vi "FPGA.vi"() -> ()   [LabVIEW 2015]
uses:
  Controls/HID Data.ctl
  <vilib>/userdefined/High Color/IMAQdx.ctl
  <vilib>/vision/Image Controls.llb/IMAQ Image.ctl
  Controls/HID State.ctl
  Controls/FGV_Options.ctl
  <vilib>/nisyscfg/Close (System).vi
  <vilib>/nisyscfg/nisyscfg.lvlib
  <resource>/objmgr/motionsysapi.rc
panel:
  out "TXT_002":string
  in  "LBL_010":u16(ring) caption="FPGA Target" items=["Select your device..."]
  in  "LBL_009":path caption="FPGA Bitfile Path"
  in  "BOOL_004":bool
  in  "BOOL_003":bool
  in  "LBL_012":u16=1 caption="FIFO Timer (mS)"
  in  "LBL_013":u8=100 caption="Memory Writer Timer (uS)"
  in  "LBL_011":u32=1000 caption="Row Timer (uS)"
  # "FPGA Taget Settings"
  # "FPGA Timing Settings"
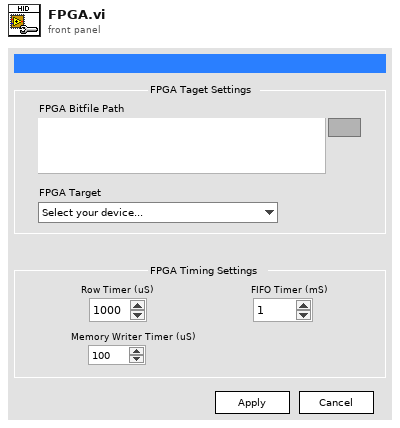
[diagram p1: front panel]
types:
  T1 = typedef "FGV_Options.ctl" = enum16{"Read from File", "Write to File", "Get", "Set"}
  T2 = cluster{"FPGA Alias":string, "FPGA Bitfile":path, "Found Aliases":string[]}
  T3 = typedef "HID Data.ctl" = cluster{"IMAQdx Session":T4, "Resampled Image":T5, "Low Level Grab":T5, "X Resolution":i32, "Y Resolution":i32, "Image Threshold":u8, "Reset Value":i32, "FIFO Timer":u16, "Row Timer":u32, "Memory Writer Timer":u8, "Color":enum16{"Green", "Blue", "Red", "White", "Pink", "Yellow", "Turquoise", "Black"}, "Top":bool[][], "Bottom":bool[][], "Timeout (ms)":i32, "Menu Tag":string, "Color Background":enum16{"Green", "Blue", "Red", "White", "Pink", "Yellow", "Turquoise", "Black"}, "FPGA VI Reference":refnum<k20>, "Next Steps":T6[], "Turn off LED Matrix":bool, "FPGA Alias":string, "FPGA Bitfile":path, "Localized Texts":cluster{"Status Text":cluster{"Status Text Table":string[], "Status Text Index":i32}, "Controls":cluster{"Control Text Table":string[], "Control Text Index":i32}, "Titles":cluster{"Titles Text Table":string[], "Titles Text Index":i32}}, "Language":u16}
  T4 = typedef "IMAQdx.ctl" = refnum<k21>
  T5 = typedef "IMAQ Image.ctl" = refnum<image>
  T6 = typedef "HID State.ctl" = enum16{"Initialize", "Set FPGA Parametes", "Set Camera Parameters", "Set LED Matrix Parameters", "Initialize FPGA Interface", "Initialize Camera", "Start FPGA VI", "Start Camera", "Wait for Event", "Update UI", "Acquire", "Process Image", "Get Boolean Arrays", "Send to FPGA", "Menu Pop-Up", "Menu Actions", "Handle Errors", "Close Camera", "Close FPGA", "Stop", "Exit"}
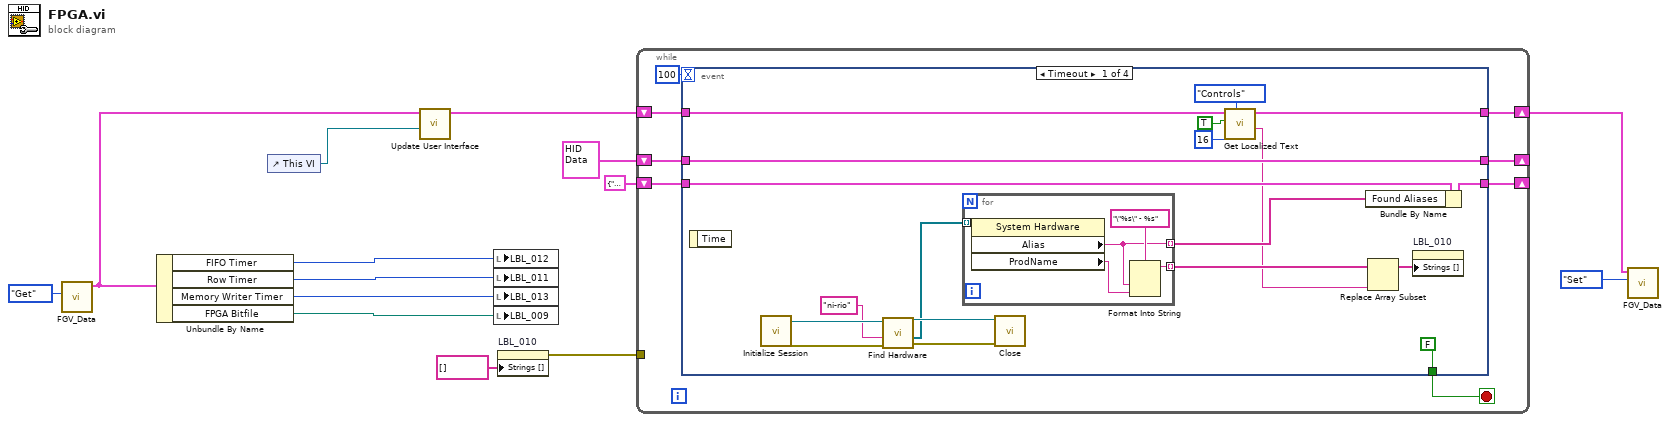
[diagram p0: block diagram]
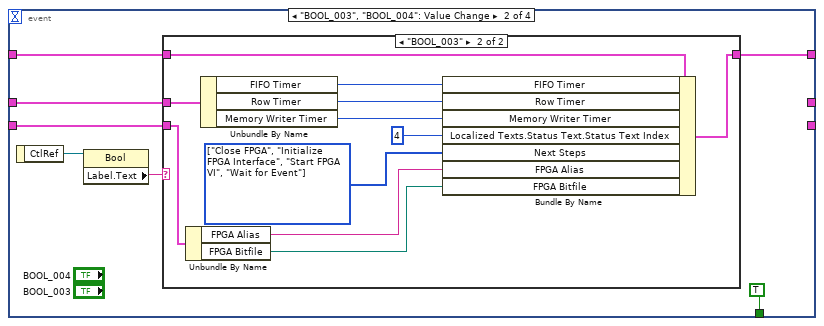
[diagram p2: hidden frame]
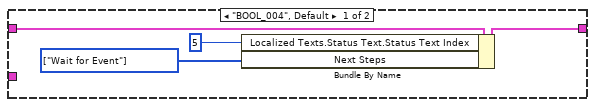
[diagram p3: hidden frame]
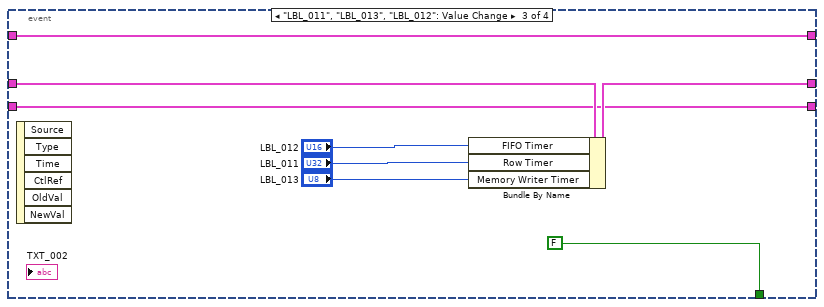
[diagram p4: hidden frame]
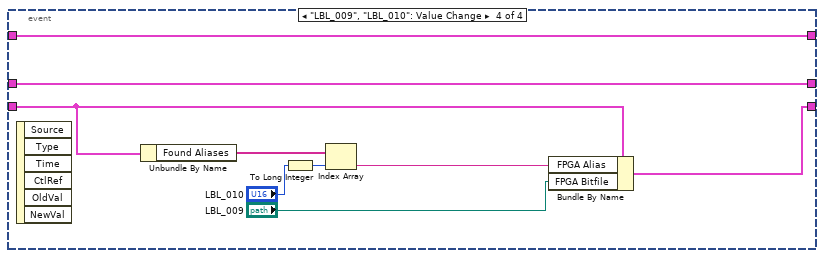
[diagram p5: hidden frame]
diagram:
  n1 = call "FGV_Data.vi"("Option"=FGV_Options."Get") -> ("Data Out"=w3:T3)  [unwired: 9 in, 1 out]
  n2 = Unbundle By Name(w3) -> ("FIFO Timer"=w9:u16, "Row Timer"=w8:u32, "Memory Writer Timer"=w7:u8, "FPGA Bitfile"=w6:path)
  n3 = control-ref of="This VI"() -> (w4:refnum<vi>)
  n4 = call "Update User Interface.vi"("VI Refnum"=w4, "Data In"=w3) -> ("Data Out"=w5:T3)  [unwired: 8 in, 1 out]
  n5 = local write "LBL_012"(w9) -> ()
  n6 = local write "LBL_011"(w8) -> ()
  n7 = local write "LBL_013"(w7) -> ()
  n8 = local write "LBL_009"(w6) -> ()
  n9 = property on="LBL_010" class="Ring (strict)"("Strings []"=string[] []) -> (error out=w1:errorcluster)  [unwired: 2 in, 1 out]
  n10 = while {
    shift-right: [w22] -> w10
    shift-left: w5 -> [w21]
    shift-right: [w18] -> _
    shift-left: T3 {"IMAQdx Session"="", "Resampled Image"=refnum, "Low Level Grab"=refnum, "X Resolution"=0, "Y Resolution"=0, "Image Threshold"=0, "Reset Value"=0, "FIFO Timer"=0, "Row Timer"=0, "Memory Writer Timer"=0, "Color"=enum."Red", "Top"=array32x96[3072 elements], "Bottom"=array32x96[3072 elements], "Timeout (ms)"=0, "Menu Tag"="", "Color Background"=enum."White", "FPGA VI Reference"=refnum, "Next Steps"=[], "Turn off LED Matrix"=FALSE, "FPGA Alias"="", "FPGA Bitfile"=path "", "Localized Texts"={"Status Text"={"Status Text Table"=[], "Status Text Index"=0}, "Controls"={"Control Text Table"=[], "Control Text Index"=0}, "Titles"={"Titles Text Table"=[], "Titles Text Index"=0}}, "Language"=0} ("Data In TMP") -> [w19]
    shift-right: [w15] -> _
    shift-left: T2 {"FPGA Alias"="PXI1Slot2", "FPGA Bitfile"=path "C:/Users/PXI-MKT/Desktop/2016_03_17_Hand Illuminator Demo/Hand Illuminator Demo/FPGA Bitfiles/HandIlluminatorD_FPGATarget_FPGAFINALv2_pLmkY6Ey6Qk.lvbitx", "Found Aliases"=[]} -> [w16]
    tunnel: w1 -> [_]
    stop <- w20 stop-if-true
    n11 = event shown="[0] Timeout" {
      selector: _ -> [_ _ _ _]
      dyn-events: _ -> [_ _ _ _]
      timeout: 100 -> [_ _ _ _]
      tunnel: [w24 w50 w76 w85] -> w22
      tunnel: w21 -> [w25 w51 w76 w85]
      tunnel: [FALSE TRUE FALSE _] -> w20
      tunnel: w19 -> [w41 w48 w75 w84]
      tunnel: [w41 _ w74 w84] -> w18
      tunnel: [w32 _ w69 w80] -> w15
      tunnel: w16 -> [w33 w47 w69 w83]
      event Timeout {
        n12 = event-data() -> ()  [unwired: 1 in, 1 out]
        n13 = call <vilib>:"Initialize Session.vi"() -> ("error out"=w39:errorcluster, "Session out"=w37:refnum<k21>)  [unwired: 10 in]
        n14 = call <vilib>:"Find Hardware.vi"("error in (no error)"=w39, "Experts"="ni-rio", "Session in"=w37) -> ("error out"=w38:errorcluster, "Resources out"=w34:refnum<k20>[], "Session out"=w36:refnum<k21>)  [unwired: 5 in, 1 out]
        n15 = for {
          tunnel: w34 -> [w46] mode=indexing
          tunnel: [w43] -> w31 mode=indexing
          tunnel: [w42] -> w30 mode=indexing
          n16 = property class="System Hardware"(reference=w46) -> ("Alias"=w43:string, "ProdName"=w44:string)  [unwired: 1 in, 2 out]
          n17 = Format Into String(format string="\"%s\" - %s", w43, w44) -> (resulting string=w42:string)  [unwired: 2 in, 1 out]
        }
        n18 = call-poly <vilib>:"Close.vi"("error in (no error)"=w38, "Session in"=w36) -> ()  [unwired: 9 in, 1 out]
        n19 = call "Get Localized Text.vi"("Text Type"=enum16{"Status", "Title", "Controls"}."Controls", "Text Index"=16, "Force Index"=TRUE, "Data In"=w25) -> ("Localized Text"=w23:string, "Data Out"=w24:T3)  [unwired: 6 in]
        n20 = Bundle By Name(cluster=w33, "Found Aliases"=w31) -> (w32:T2)
        n21 = Replace Array Subset(array=w30, new element=w23) -> (w29:string[])  [unwired: 1 in]
        n22 = property on="LBL_010" class="Ring (strict)"("Strings []"=w29) -> ()  [unwired: 2 in, 2 out]
      }
      event "BOOL_003", "BOOL_004": Value Change {
        n23 = event-data() -> ("CtlRef"=w52:refnum<vi>)  [unwired: 1 in]
        n24 = property class="Bool"(reference=w52) -> ("Label.Text"=w49:string)  [unwired: 1 in, 2 out]
        n25 = case shown="\"BOOL_003\"" w49 {
          tunnel: w51 -> [w57 w68]
          tunnel: [w56 w67] -> w50
          tunnel: w48 -> [_ w66]
          tunnel: w47 -> [_ w61]
          frame "BOOL_004", Default {
            w55 = T6[] [enum."Wait for Event"] items=["Initialize", "Set FPGA Parametes", "Set Camera Parameters", "Set LED Matrix Parameters", "Initialize FPGA Interface", "Initialize Camera", "Start FPGA VI", "Start Camera", "Wait for Event", "Update UI", "Acquire", "Process Image", "Get Boolean Arrays", "Send to FPGA", "Menu Pop-Up", "Menu Actions", "Handle Errors", "Close Camera", "Close FPGA", "Stop", "Exit"] ("Array")
            n26 = Bundle By Name(cluster=w57, "Localized Texts.Status Text.Status Text Index"=5 ("Status"), "Next Steps"=w55) -> (w56:T3)
          }
          frame "BOOL_003" {
            w62 = T6[] [enum."Close FPGA", enum."Initialize FPGA Interface", enum."Start FPGA VI", enum."Wait for Event"] items=["Initialize", "Set FPGA Parametes", "Set Camera Parameters", "Set LED Matrix Parameters", "Initialize FPGA Interface", "Initialize Camera", "Start FPGA VI", "Start Camera", "Wait for Event", "Update UI", "Acquire", "Process Image", "Get Boolean Arrays", "Send to FPGA", "Menu Pop-Up", "Menu Actions", "Handle Errors", "Close Camera", "Close FPGA", "Stop", "Exit"] ("Array")
            n27 = Unbundle By Name(w61) -> ("FPGA Alias"=w60:string, "FPGA Bitfile"=w59:path)
            n28 = Unbundle By Name(w66) -> ("FIFO Timer"=w65:u16, "Row Timer"=w64:u32, "Memory Writer Timer"=w63:u8)
            n29 = Bundle By Name(cluster=w68, "FIFO Timer"=w65, "Row Timer"=w64, "Memory Writer Timer"=w63, "Localized Texts.Status Text.Status Text Index"=4 ("Status"), "Next Steps"=w62, "FPGA Alias"=w60, "FPGA Bitfile"=w59) -> (w67:T3)
          }
        }
      }
      event "LBL_011", "LBL_013", "LBL_012": Value Change {
        n30 = event-data() -> ()  [unwired: 1 in, 6 out]
        n31 = Bundle By Name(cluster=w75, "FIFO Timer"="LBL_012", "Row Timer"="LBL_011", "Memory Writer Timer"="LBL_013") -> (w74:T3)
      }
      event "LBL_009", "LBL_010": Value Change {
        n32 = event-data() -> ()  [unwired: 1 in, 6 out]
        n33 = Unbundle By Name(w83) -> ("Found Aliases"=w82:string[])
        n34 = To Long Integer(number="LBL_010") -> (32bit integer=w78:i32)
        n35 = Index Array(array=w82, index=w78) -> (element=w79:string)
        n36 = Bundle By Name(cluster=w83, "FPGA Alias"=w79, "FPGA Bitfile"="LBL_009") -> (w80:T2)
      }
    }
  }
  n37 = call "FGV_Data.vi"("Option"=FGV_Options."Set", "Data In"=w10) -> ()  [unwired: 8 in, 2 out]
